vi "Choose case dewbot 10.vi"(4 "Next FR motor value":dbl=0.6, 6 "Next BL motor value":dbl=0.6, 9 "Next BR motor value":dbl=0.6, 10 "Next FL motor value":dbl=0.6, 11 "Set Tac value":dbl) -> (0 "Last FR motor value":dbl=0.6, 1 "Last BL motor value":dbl=0.6, 2 "Last BR motor value":dbl=0.6, 3 "Last FL motor value":dbl=0.6, 5 "Next primitive?":bool)   [LabVIEW 2013]
uses:
  Begin/Global Variables.vi
  Begin/Global Refnums.vi
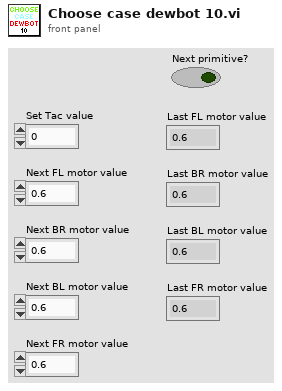
[diagram p1: front panel]
types:
  T1 = typedef "WPI_GyroDevRef.ctl" = cluster{"DevStatus":errorcluster, "Analog Module":T2, "Analog Channel":T3, "Offset":dbl, "Gain (VoltsPerDegree/Second)":dbl}
  T2 = typedef "FPGA_TypedefAnalogModule.ctl" = enum16{"Analog Module 1", "Analog Module 2"}
  T3 = typedef "FPGA_AIChannel.ctl" = enum8{"AI 1", "AI 2", "AI 3", "AI 4", "AI 5", "AI 6", "AI 7", "AI 8", "Invalid"}
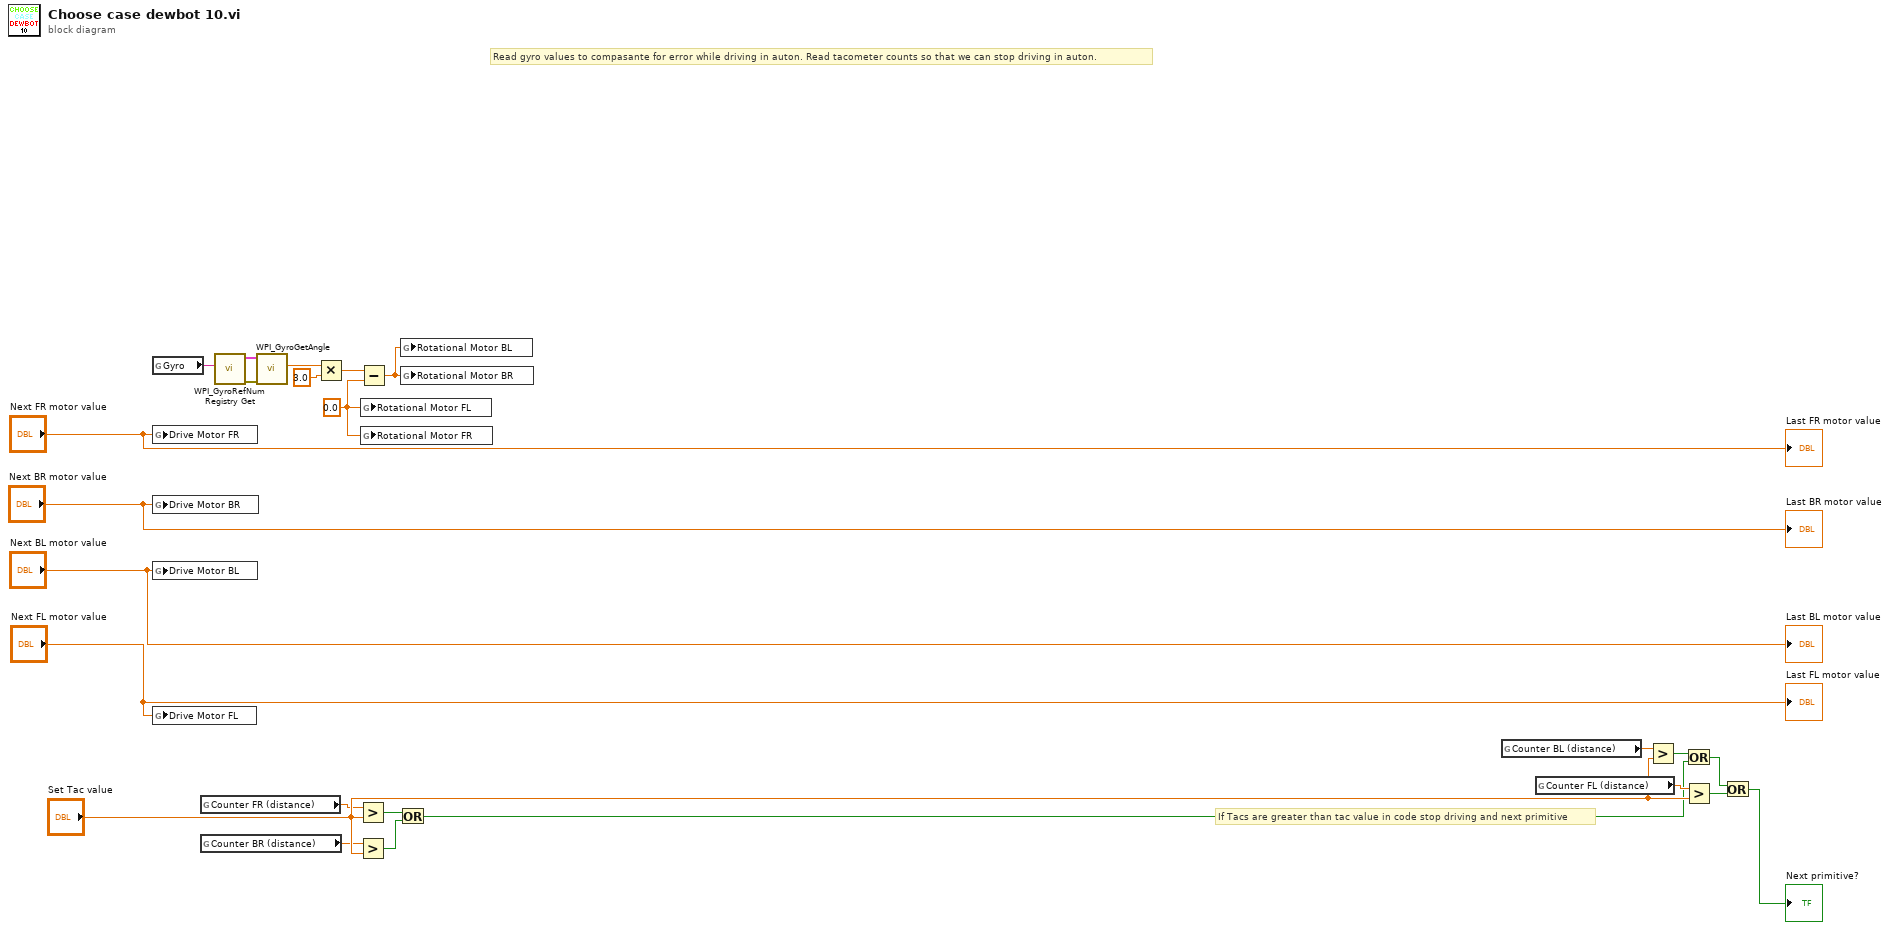
[diagram p0: block diagram]
diagram:
  w1 = 0.0 ("t")
  # "Read gyro values to compasante for error while driving in auton. Read tacometer counts so that we can stop driving in auton."
  # "If Tacs are greater than tac value in code stop driving and next primitive"
  n1 = global read "Global Refnums.vi" "Gyro"() -> (w2:string)
  n2 = global write "Global Variables.vi" "Drive Motor FR"("Next FR motor value") -> ()
  n3 = global write "Global Variables.vi" "Drive Motor BR"("Next BR motor value") -> ()
  n4 = global write "Global Variables.vi" "Drive Motor BL"("Next BL motor value") -> ()
  n5 = global write "Global Variables.vi" "Drive Motor FL"("Next FL motor value") -> ()
  n6 = global read "Global Refnums.vi" "Counter FR (distance)"() -> (w12:dbl)
  n7 = global read "Global Refnums.vi" "Counter BR (distance)"() -> (w9:dbl)
  n8 = call <vilib>:"WPI_GyroRefNum Registry Get.vi"("refnum name"=w2) -> ("error out"=w7:errorcluster, "GyroDevRef"=w6:T1)  [unwired: 9 in]
  n9 = call <vilib>:"WPI_GyroGetAngle.vi"("error in (no error)"=w7, "GyroDevRef"=w6) -> ("Angle"=w5:dbl)  [unwired: 6 in, 3 out]
  n10 = Multiply(x=w5, y=3.0) -> (x*y=w3:dbl)
  n11 = Greater?(x=w12, y="Set Tac value") -> (0:w17:bool)
  n12 = Greater?(x=w9, y="Set Tac value") -> (0:w18:bool)
  n13 = Subtract(x=w3, y=w1) -> (x-y=w8:dbl)
  n14 = global write "Global Variables.vi" "Rotational Motor FL"(w1) -> ()
  n15 = global write "Global Variables.vi" "Rotational Motor FR"(w1) -> ()
  n16 = Or(x=w17, y=w18) -> (x .or. y?=w11:bool)
  n17 = global write "Global Variables.vi" "Rotational Motor BL"(w8) -> ()
  n18 = global write "Global Variables.vi" "Rotational Motor BR"(w8) -> ()
  n19 = global read "Global Refnums.vi" "Counter BL (distance)"() -> (w14:dbl)
  n20 = global read "Global Refnums.vi" "Counter FL (distance)"() -> (w13:dbl)
  n21 = Greater?(x=w14, y="Set Tac value") -> (0:w16:bool)
  n22 = Or(x=w16, y=w11) -> (x .or. y?=w15:bool)
  n23 = Greater?(x=w13, y="Set Tac value") -> (0:w10:bool)
  n24 = Or(x=w15, y=w10) -> (x .or. y?=→"Next primitive?":bool)
  "Last BR motor value" <- "Next BR motor value"
  "Last FL motor value" <- "Next FL motor value"
  "Last FR motor value" <- "Next FR motor value"
  "Last BL motor value" <- "Next BL motor value"
